vi "logger.vi"() -> ()   [LabVIEW 2014]
panel:
  in  "message":string
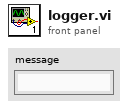
[diagram p1: front panel]
types:
  T1 = enum16{"open", "replace", "create", "open or create", "replace or create", "replace or create with confirmation"}
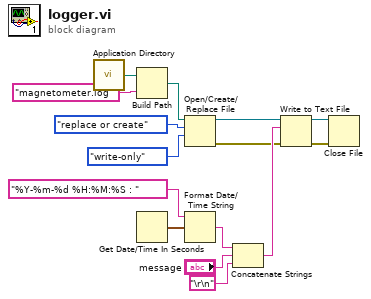
[diagram p0: block diagram]
diagram:
  n1 = call <vilib>:"Application Directory.vi"() -> ("Application Directory"=w11:path)
  n2 = Build Path(base path=w11, name or relative path="magnetometer.log") -> (appended path=w9:path)
  n3 = Get Date/Time In Seconds() -> (seconds since 1Jan1904=w12:timestamp)
  n4 = Open/Create/Replace File(file path (use dialog)=w9, operation (0:open)=T1."replace or create", access (0:read/write)=enum16{"read/write", "read-only", "write-only"}."write-only") -> (refnum out=w13:refnum<file>, error out=w1:errorcluster)  [unwired: 3 in, 1 out]
  n5 = Format Date/Time String(time format string (%c)="%Y-%m-%d %H:%M:%S : ", seconds (now)=w12) -> (date/time string=w7:string)  [unwired: 1 in]
  n6 = Concatenate Strings(w7, "message", "\r\n") -> (w4:string)
  n7 = Write to Text File(file (use dialog)=w13, text=w4, error in=w1) -> (refnum out=w2:refnum<file>, error out=w3:errorcluster)  [unwired: 1 in, 1 out]
  n8 = Close File(refnum=w2, error in=w3) -> ()  [unwired: 2 out]
